vi "ryTimerEx Custom.vi"() -> ()   [LabVIEW 2021]
uses:
  Lib/ryTimer.lvclass/ryTimer.ctl
  f249acfa-4261-438f-8338-865fe7d44341.vi
  Lib/SubVIs/ryTimer Set Properties.vi
  Lib/SubVIs/ryTimer Daemon.vi
  <vilib>/Utility/error.llb/Error Cluster From Error Code.vi
  Lib/ryTimer.lvclass
panel:
  out "Time Ellapsed (ms)":u32
  out "Error":errorcluster
  out "Custom Element":T1
  # "Custom Message \"EXIT\"\nshould be enqueue after\n5 seconds."
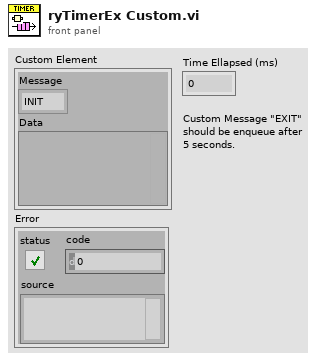
[diagram p1: front panel]
types:
  T1 = cluster{"Message":enum16{"INIT", "EXIT"}, "Data":variant}
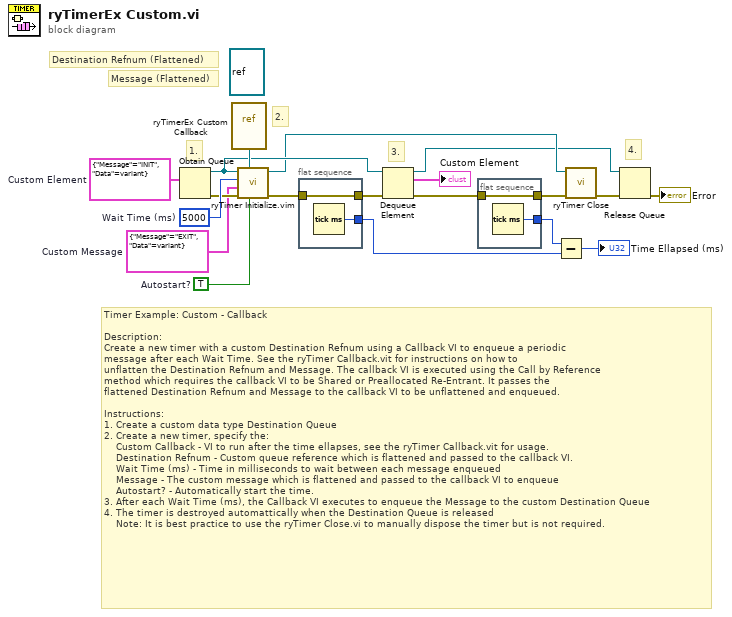
[diagram p0: block diagram]
diagram:
  (unwired) refnum<vi> refnum ("Custom Callback")
  w14 = T1 {"Message"=enum."EXIT", "Data"=variant}  # Custom Message
  w16 = T1 {"Message"=enum."INIT", "Data"=variant}  # Custom Element
  w19 = TRUE  # Autostart?
  w18 = u32 5000  # Wait Time (ms)
  # "4."
  # "2."
  # "1."
  # "3."
  # "Timer Example: Custom - Callback\n\nDescription:\nCreate a new timer with a custom Destination Refnum using a Callback VI to enqueue a periodic\nmessage after each Wait Time. See the ryTimer Callback.vit for instructions on how to\nunflatten the Destination Refnum and Message. The callback VI is executed using the Call by Reference\nmethod which requires the callback VI to be Shared or Preallocated Re-Entrant. It passes the\nflattened Destination Refnum and Message to the callback VI to be unflattened and enqueued.\n\nInstructions:\n1. Create a custom data type Destination Queue\n2. Create a new timer, specify the:\n    Custom Callback - VI to run after the time ellapses, see the ryTimer Callback.vit for usage.\n    Destination Refnum - Custom queue reference which is flattened and passed to the callback VI.\n    Wait Time (ms) - Time in milliseconds to wait between each message enqueued\n    Message - The custom message which is flattened and passed to the callback VI to enqueue\n    Autostart? - Automatically start the time.\n3. After each Wait Time (ms), the Callback VI executes to enqueue the Message to the custom Destination Queue\n4. The timer is destroyed automattically when the Destination Queue is released\n    Note: It is best practice to use the ryTimer Close.vi to manually dispose the timer but is not required."
  # "Message (Flattened)"
  # "Destination Refnum (Flattened)"
  n1 = Obtain Queue(element data type=w16) -> (queue out=w13:refnum<queue>, error out=w17:errorcluster)  [unwired: 4 in, 1 out]
  n2 = vi-ref "ryTimerEx Custom Callback.vi"() -> (w15:refnum<vi>)
  n3 = call "ryTimer Initialize.vim"("Autostart? (F)"=w19, "Custom Callback"=w15, "error in (no error)"=w17, "Message"=w14, "Wait Time (ms)"=w18, "Destination Refnum [Q,UE,Any]"=w13) -> ("error out"=w6:errorcluster, "Timer out"=w11:refnum<class "ryTimer.lvclass">)  [unwired: 4 in]
  n4 = flat-sequence {
    tunnel: [w21] -> w7
    tunnel: w6 -> [w21]
    tunnel: [w20] -> w2
    frame #0 {
      n5 = Tick Count (ms)() -> (millisecond timer value=w20:u32)
    }
  }
  n6 = Dequeue Element(queue=w13, error in (no error)=w7) -> (queue out=w9:refnum<queue>, element=→"Custom Element":T1, error out=w5:errorcluster)  [unwired: 1 in, 1 out]
  n7 = flat-sequence {
    tunnel: [w23] -> w4
    tunnel: w5 -> [w23]
    tunnel: [w22] -> w3
    frame #0 {
      n8 = Tick Count (ms)() -> (millisecond timer value=w22:u32)
    }
  }
  n9 = Subtract(x=w3, y=w2) -> (x-y=→"Time Ellapsed (ms)":u32)
  n10 = call "ryTimer Close.vi"("error in (no error)"=w4, "Timer in"=w11) -> ("error out"=w10:errorcluster)  [unwired: 9 in]
  n11 = Release Queue(queue=w9, error in (no error)=w10) -> (error out=→"Error":errorcluster)  [unwired: 1 in, 2 out]
